vi "Agilent MXA Series Acquire Trace.vi"() -> ()   [LabVIEW 2018]
doc: "This example shows how to configure the spectrum analyzer to acquire a trace."
uses:
  Public/Configure/Configure Frequency (Start Stop).vi
  Public/Configure/Configure Level (Normal).vi
  Agilent MXA Series.lvlib
panel:
  in  "Manual Detector Type (0: Normal)":i32(ring) items=["Normal", "Average", "Peak", "Sample", "Negative peak"]
  in  "Timeout (50000 ms)":i32=50000 format="%.0g"
  in  "Trace Type (0: Clear Write)":i32(ring) items=["Clear Write", "Average", "Maximum Hold", "Minimum Hold"]
  in  "Trace Name (1: Trace 1)":i32(ring)=1 items=["Trace 1"=1, "Trace 2"=2, "Trace 3"=3, "Trace 4"=4]
  out "Trace Waveform":cluster{"X Array":dbl[], "Y Array":dbl[]}(graph)
  in  "Reference Level Offset (0 dB)":dbl
  in  "Reference Level (10 dBm)":dbl=10.0
  in  "Input Impedance (0: 50 ohms)":i32(ring) items=["50", "75"]
  in  "Stop Frequency (25 E+9 Hz)":dbl=25000000000.0
  in  "Start Frequency (100 E+3 Hz)":dbl=100000.0
  in  "VISA resource name":refnum<visa-resource-name>
  # "(c) 2007-2015 National Instruments.  ALL RIGHTS RESERVED."
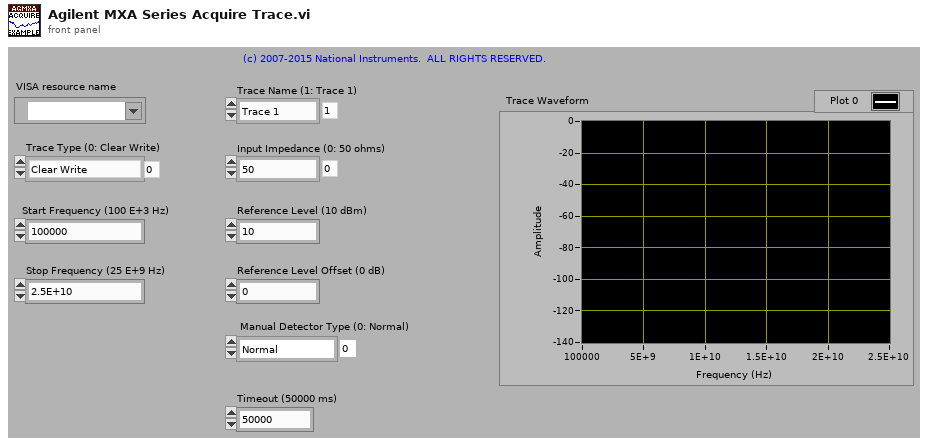
[diagram p1: front panel]
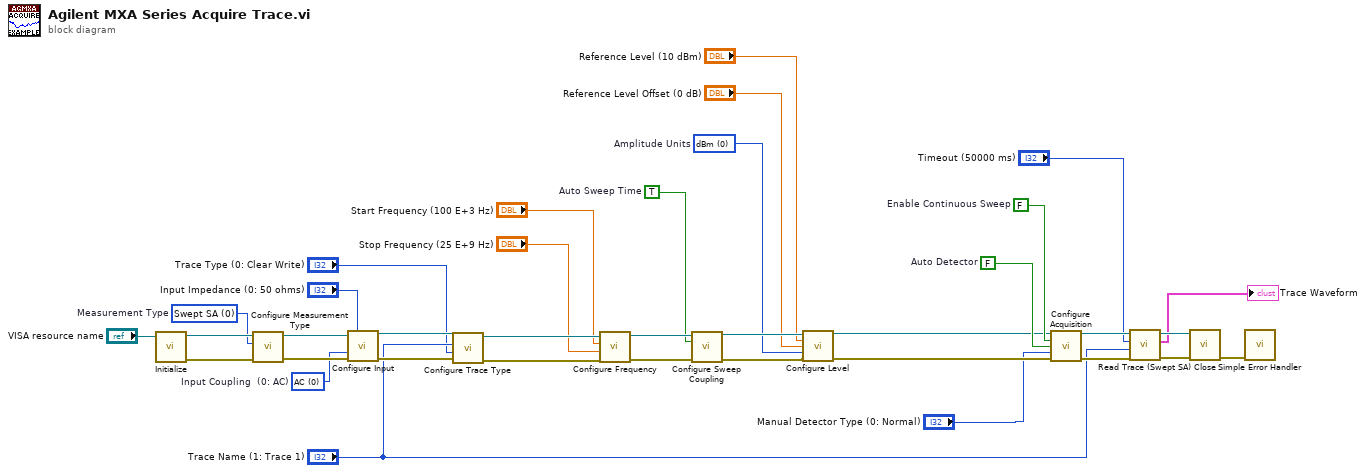
[diagram p0: block diagram]
diagram:
  w14 = 0 items=["AC", "DC"]  # Input Coupling  (0: AC)
  w22 = 0 items=["Swept SA", "Channel Power", "Occupied Bandwidth", "Power Stat CCDF", "Adjacent Channel Power", "Burst Power", "Spurious Emissions", "Spectrum Emission Mask", "List Sweep"]  # Measurement Type
  w21 = TRUE  # Auto Sweep Time
  w20 = FALSE  # Auto Detector
  w19 = FALSE  # Enable Continuous Sweep
  w4 = 0 items=["dBm", "dBV", "dBmV", "dBuV", "Volts", "Watts"]  # Amplitude Units
  n1 = call "Initialize.vi"("VISA resource name"="VISA resource name") -> ("error out"=w27:errorcluster, "VISA resource name out"=w28:refnum<visa-resource-name>)  [unwired: 9 in]
  n2 = call "Configure Measurement Type.vi"("error in (no error)"=w27, "Measurement Type (0: Swept SA)"=w22, "VISA resource name"=w28) -> ("error out"=w15:errorcluster, "VISA resource name out"=w18:refnum<visa-resource-name>)  [unwired: 7 in]
  n3 = call "Configure Input.vi"("VISA resource name"=w18, "Input Impedance (0: 50 ohms)"="Input Impedance (0: 50 ohms)", "Input Coupling  (0: AC)"=w14, "error in (no error)"=w15) -> ("VISA resource name out"=w17:refnum<visa-resource-name>, "error out"=w16:errorcluster)  [unwired: 10 in]
  n4 = call "Configure Trace Type.vi"("error in (no error)"=w16, "Trace Type (0: Clear Write)"="Trace Type (0: Clear Write)", "Trace Name (1: Trace 1)"="Trace Name (1: Trace 1)", "VISA resource name"=w17) -> ("error out"=w31:errorcluster, "VISA resource name out"=w32:refnum<visa-resource-name>)  [unwired: 6 in]
  n5 = call-poly "Configure Frequency.vi"("error in (no error)"=w31, "Stop Frequency (2.65E+10 Hz)"="Stop Frequency (25 E+9 Hz)", "Start Frequency (1E+7 Hz)"="Start Frequency (100 E+3 Hz)", "VISA resource name"=w32) -> ("error out"=w25:errorcluster, "VISA resource name out"=w26:refnum<visa-resource-name>)  [unwired: 6 in]
  n6 = call "Configure Sweep Coupling.vi"("VISA resource name"=w26, "Auto Sweep Time (T: Enable)"=w21, "error in (no error)"=w25) -> ("VISA resource name out"=w8:refnum<visa-resource-name>, "error out"=w11:errorcluster)  [unwired: 11 in]
  n7 = call-poly "Configure Level.vi"("VISA resource name"=w8, "Reference Level (0 dBm)"="Reference Level (10 dBm)", "Reference Level Offset (0 dB)"="Reference Level Offset (0 dB)", "Amplitude Units (0: dBm)"=w4, "error in (no error)"=w11) -> ("VISA resource name out"=w9:refnum<visa-resource-name>, "error out"=w10:errorcluster)  [unwired: 9 in]
  n8 = call "Configure Acquisition.vi"("VISA resource name"=w9, "Enable Continuous Sweep (T: Enable)"=w19, "Auto Detector (T: Enable)"=w20, "Manual Detector Type (0: Normal)"="Manual Detector Type (0: Normal)", "error in (no error)"=w10) -> ("VISA resource name out"=w24:refnum<visa-resource-name>, "error out"=w23:errorcluster)  [unwired: 9 in]
  n9 = call "Read Trace (Swept SA).vi"("error in (no error)"=w23, "Trace Name (1: Trace 1)"="Trace Name (1: Trace 1)", "Timeout (10000 ms)"="Timeout (50000 ms)", "VISA resource name"=w24) -> ("error out"=w34:errorcluster, "Trace Waveform"=→"Trace Waveform":cluster{"X Array":dbl[], "Y Array":dbl[]}, "VISA resource name out"=w36:refnum<visa-resource-name>)  [unwired: 5 in]
  n10 = call "Close.vi"("error in (no error)"=w34, "VISA resource name"=w36) -> ("error out"=w35:errorcluster)  [unwired: 9 in]
  n11 = call <vilib>:"Simple Error Handler.vi"("error in (no error)"=w35) -> ()  [unwired: 4 in, 5 out]
